vi "XIPIN_Digital_Pre-Distortion_6_0.vi"   [LabVIEW 2017]
doc: "Digital Pre-Distortion(DPD) is an important component in the signal processing chains of many wireless communications systems. The Xilinx DPD LogiCORE provides users an off-the-shelf means to integrate this functionality in their digital radio front end(DFE) design for a range of wireless interface standards based on system-level parameters. The core implementation is delivered through the Xilinx CORE Generator system, and is designed to take advantage of the advanced features of Xilinx FPGA devices.\n------------------------------------\n<b>Need License</b> : Yes\n<b>Interface</b> : AXI4-Stream AXI4-Lite"
uses:
  <vilib>/rvi/XilinxIP/XIPIN_XNode/niFpgaXIPIN.xnode
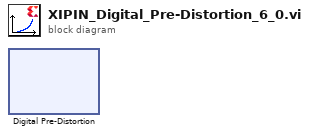
[diagram p0: block diagram]
diagram:
  n1 = xnode ("Digital Pre-Distortion")() -> ()
